vi "Populate_Do.vi"(8 "error in (no error)":errorcluster, 9 "Value":string, 10 "Lower case name":string, 11 "Run System Exec in":refnum<class "Run System Exec.lvclass">) -> (0 "error out":errorcluster, 1 "Success?":bool, 3 "Run System Exec out":refnum<class "Run System Exec.lvclass">)   [LabVIEW 2020, in "ProjectBuilder.lvlib" / "Run System Exec.lvclass"]
doc: "Override to populate private data from strings.\n\nThis implementation can set the \"alias\", \"command line\" and \"standard input\" strings, the \"working directory\" path, the \"expected output size\" number and the \"skip prefic cmd\" boolean."
uses:
  Run System Exec.lvclass
  C:/Current projects/WS/LV32.2020..ProjectBuilder/Class/Project Action/Project Action.lvclass
  Run System Exec.lvclass/Run System Exec.ctl
  Project Action/Project Action.lvclass/Project Action.ctl
  ProjectBuilder.lvlib
  Project Action/Project Action.lvclass
  PPL/HDH.ClassLoader.lvlibp
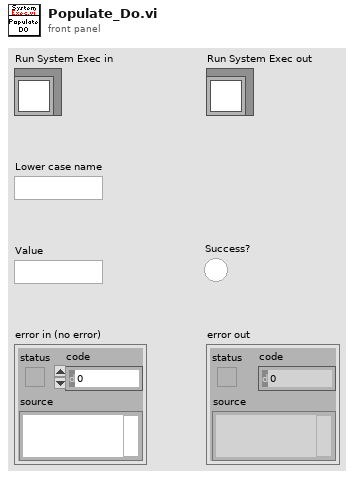
[diagram p1: front panel]
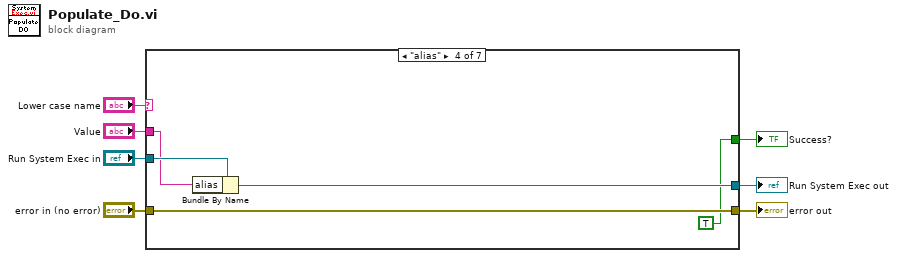
[diagram p0: block diagram]
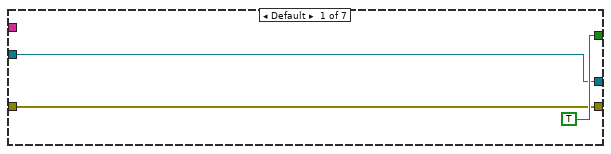
[diagram p2: hidden frame]
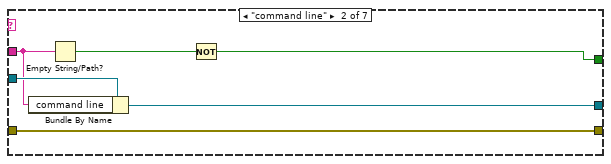
[diagram p3: hidden frame]
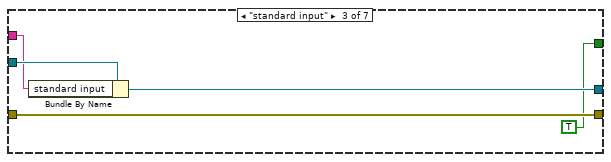
[diagram p4: hidden frame]
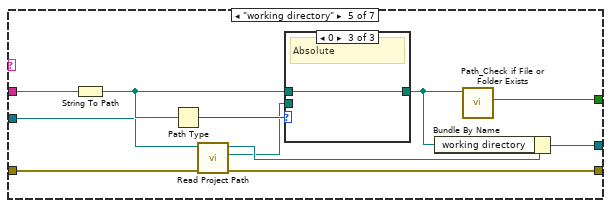
[diagram p5: hidden frame]
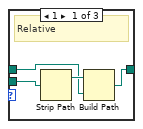
[diagram p6: hidden frame]
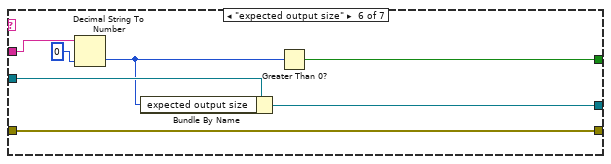
[diagram p8: hidden frame]
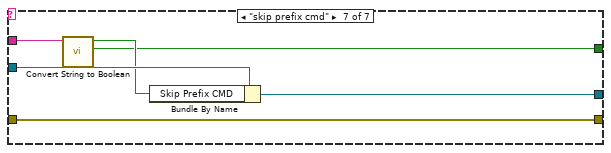
[diagram p9: hidden frame]
diagram:
  n1 = case shown="\"alias\"" "Lower case name" {
    tunnel: [TRUE w12 TRUE TRUE w27 w43 w51] -> w6
    tunnel: [w9 w15 w20 w25 w37 w48 w54] -> w5
    tunnel: "Run System Exec in" -> [w9 w16 w21 w26 w31 w49 w55]
    tunnel: [w8 w11 w18 w23 w33 w47 w50] -> w3
    tunnel: "error in (no error)" -> [w8 w11 w18 w23 w32 w47 w50]
    tunnel: "Value" -> [_ w14 w19 w24 w36 w46 w53]
    frame Default {
    }
    frame "command line" {
      n2 = Bundle By Name(cluster=w16, "command line"=w14) -> (w15:refnum<class "Run System Exec.lvclass">)
      n3 = Empty String/Path?(string/path=w14) -> (empty?=w13:bool)
      n4 = Not(x=w13) -> (.not. x?=w12:bool)
    }
    frame "standard input" {
      n5 = Bundle By Name(cluster=w21, "standard input"=w19) -> (w20:refnum<class "Run System Exec.lvclass">)
    }
    frame "alias" {
      n6 = Bundle By Name(cluster=w26, "alias"=w24) -> (w25:refnum<class "Run System Exec.lvclass">)
    }
    frame "working directory" {
      n7 = String To Path(string=w36) -> (path=w34:path)
      n8 = Path Type(1:w34) -> (0:w35:i16)
      n9 = call "Read Project Path.vi"("error in (no error)"=w32, "Project Action in"=w31) -> ("error out"=w33:errorcluster, "Project Path"=w29:path, "Project Action out"=w30:refnum<class "Run System Exec.lvclass">)  [unwired: 7 in]
      n10 = case shown="0" w35 {
        tunnel: [w38 _ w42] -> w28
        tunnel: w34 -> [w39 _ w42]
        tunnel: w29 -> [w41 _ _]
        frame 1 {
          # "Relative"
          n11 = Strip Path(path=w41) -> (stripped path=w40:path)  [unwired: 1 out]
          n12 = Build Path(base path=w40, name or relative path=w39) -> (appended path=w38:path)
        }
        frame Default {
          # "Not a path"
        }
        frame 0 {
          # "Absolute"
        }
      }
      n13 = Bundle By Name(cluster=w30, "working directory"=w28) -> (w37:refnum<class "Run System Exec.lvclass">)
      n14 = call "Path_Check if File or Folder Exists.vi"("File or Folder Path in"=w28) -> ("File or Folder Found?"=w27:bool)  [unwired: 9 in, 1 out]
    }
    frame "expected output size" {
      n15 = Decimal String To Number(string=w46, default (0L)=u32 0 ("default (0 I32)")) -> (number=w44:u32)  [unwired: 1 in, 1 out]
      n16 = Bundle By Name(cluster=w49, "expected output size"=w44) -> (w48:refnum<class "Run System Exec.lvclass">)
      n17 = Greater Than 0?(x=w44) -> (x > 0?=w43:bool)
    }
    frame "skip prefix cmd" {
      n18 = call "Convert String to Boolean.vi"("String"=w53) -> ("Valid string?"=w51:bool, "Boolean value"=w52:bool)  [unwired: 9 in]
      n19 = Bundle By Name(cluster=w55, "Skip Prefix CMD"=w52) -> (w54:refnum<class "Run System Exec.lvclass">)
    }
  }
  "error out" <- w3
  "Run System Exec out" <- w5
  "Success?" <- w6
